vi "F Dwf Enum Device Name.vi"(8 "error in (no error)":errorcluster, 10 "szDeviceName":string, 11 "idxDevice":i32) -> (0 "error out":errorcluster, 2 "szDeviceName out":string, 3 "function return":i32)   [LabVIEW 2024, in "Olasdwf.lvlib"]
doc: "DWFAPI int FDwfEnumDeviceName(int idxDevice, char szDeviceName[32]);"
uses:
  Olasdwf.lvlib
  Windows/System32/dwf.dll
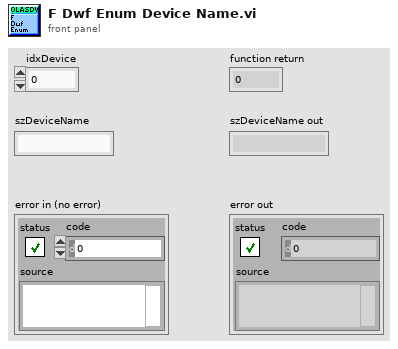
[diagram p1: front panel]
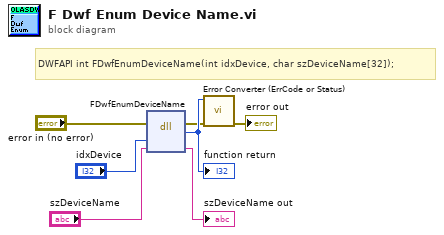
[diagram p0: block diagram]
diagram:
  # "DWFAPI int FDwfEnumDeviceName(int idxDevice, char szDeviceName[32]);"
  n1 = dll-call lib="/Windows/System32/dwf.*" fn="FDwfEnumDeviceName"(error in="error in (no error)", "idxDevice"="idxDevice", "szDeviceName"="szDeviceName") -> (error out=w2:errorcluster, w7:i32, "szDeviceName"=→"szDeviceName out":string)  [unwired: 3 in, 1 out]
  "function return" <- w7
  n2 = call "Error Converter (ErrCode or Status).vi"("error in (no error)"=w2, "error code"=w7) -> ("error out"=→"error out":errorcluster)  [unwired: 9 in]
